vi "Initialize.vi"(8 "error in":errorcluster, 10 "Device":string) -> (0 "error out":errorcluster, 3 "Flash Utility out":refnum<class "Flash Utility.lvclass">)   [LabVIEW 2018, in "Flash Utility.lvlib" / "Flash Utility.lvclass"]
uses:
  Flash Utility.lvclass
  Flash Utility.lvclass/Flash Utility.ctl
  builds/Configuration.lvlibp/Configuration.lvclass
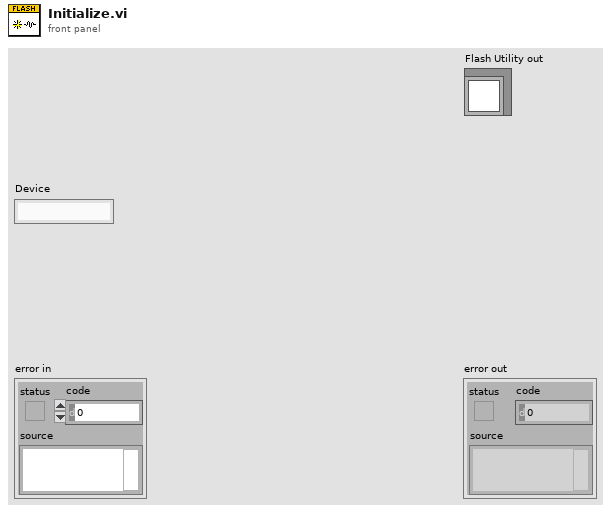
[diagram p1: front panel]
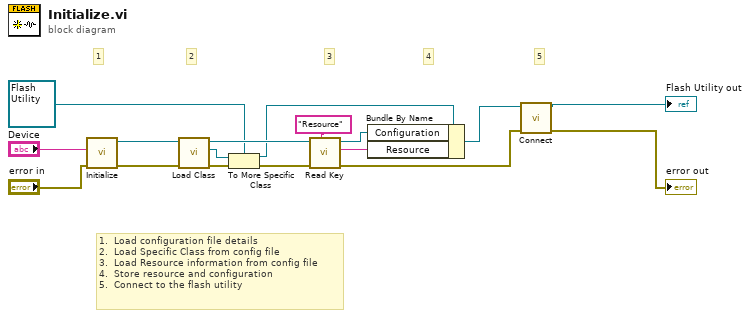
[diagram p0: block diagram]
diagram:
  # "1.  Load configuration file details\n2.  Load Specific Class from config file\n3.  Load Resource information from config file\n4.  Store resource and configuration\n5.  Connect to the flash utility"
  # "5"
  # "4"
  # "3"
  # "2"
  # "1"
  n1 = call "Initialize.vi"("error in"="error in", "Device"="Device") -> ("error out"=w3:errorcluster, "Configuration out"=w4:refnum<class "Configuration.lvclass">)  [unwired: 8 in]
  n2 = call "Load Class.vi"("error in"=w3, "Configuration in"=w4) -> ("error out"=w14:errorcluster, "Class out"=w15:refnum<class>, "Configuration out"=w13:refnum<class "Configuration.lvclass">)  [unwired: 7 in]
  n3 = To More Specific Class(target class=refnum<class "Flash Utility.lvclass"> refnum ("Flash Utility in"), reference=w15, error in=w14) -> (specific class reference=w10:refnum<class "Flash Utility.lvclass">, error out=w11:errorcluster)
  n4 = call "Read Key.vi"("Key:"="Resource", "error in"=w11, "Configuration in"=w13) -> ("error out"=w6:errorcluster, "Value"=w8:string, "Configuration out"=w9:refnum<class "Configuration.lvclass">)  [unwired: 6 in]
  n5 = Bundle By Name(cluster=w10, "Configuration"=w9, "Resource"=w8) -> (w7:refnum<class "Flash Utility.lvclass">)
  n6 = call-dynamic "Connect.vi"("error in (no error)"=w6, "Flash Utility in"=w7) -> ("error out"=→"error out":errorcluster, "Flash Utility out"=→"Flash Utility out":refnum<class "Flash Utility.lvclass">)  [unwired: 8 in]
